vi "Main.vi"(11 "Module Admin":refnum<class "Delacor_lib_QMH_Cloneable Module Admin.lvclass">) -> ()   [LabVIEW 2020, in "TDS1002 Oscilloscope.lvlib"]
doc: "This template is based off of the Queued Message Handler design pattern and the Queued Message Handler project template that ships with LabVIEW.\n\nThe main difference is that the queue is private to this module and communication between modules is performed via Broadcast and Request events.\n\nRequest events are wrapped in public API methods and are handled in the Event Handling Loop (EHL) of this VI. Any module can register for Broadcast events sent by this module. The EHL generates messages based on user interface actions.\n\nThe Message Handling Loop (MHL) processes messages generated by the EHL, or by other messages. The messages are string values, so new messages can be added easily to the Message Cases case structure in the MHL. Each message cluster can also provide an optional value for Message Data, which is a variant that can be converted to whatever message-specific data is required.\n_____\nBased on DQMH Project Template 6.1.0.94.\n____\nPantherLAB Templates 1.0.0.1\nCopyright (c) 2022, PantherLAB\n____\nPantherLAB Templates 1.0.0.5\nCopyright (c) 2022, PantherLAB"
uses:
  TDS1002 Oscilloscope.lvlib
  <vilib>/Delacor/Delacor QMH/Libraries/Cloneable Module Admin_class/Delacor_lib_QMH_Cloneable Module Admin.lvclass
  C:/Program Files (x86)/National Instruments/LabVIEW 2020/vi.lib/Delacor/Delacor QMH/Libraries/Module Admin_class/Delacor_lib_QMH_Module Admin.lvclass
  Module Data--cluster.ctl
  <vilib>/Delacor/Delacor QMH/Libraries/Cloneable Module Admin_class/Delacor_lib_QMH_Cloneable Module Admin.lvclass/Delacor_lib_QMH_Cloneable Module Admin.ctl
  Helper Loop Status--enum.ctl
  <vilib>/Delacor/Delacor QMH/Libraries/Message Queue_class/Delacor_lib_QMH_Message Queue.lvclass/Delacor_lib_QMH_Message Queue.ctl
  Stop Argument--cluster.ctl
  <vilib>/Delacor/Delacor QMH/Libraries/Module Admin_class/Delacor_lib_QMH_Module Admin.lvclass/Delacor_lib_QMH_Module Admin.ctl
  Draw Panel into Subpanel Argument--cluster.ctl
  Remove Panel from Subpanel Argument--cluster.ctl
  Connect Argument--cluster.ctl
  Disconnect Argument--cluster.ctl
  Configure acquisition Argument--cluster.ctl
  Support/Channel configuration--cluster.ctl
  Configure trigger Argument--cluster.ctl
  Trigger config--cluster.ctl
  Send software trigger Argument--cluster.ctl
  Start continuous acquistion Argument--cluster.ctl
  Stop continuous acquisition Argument--cluster.ctl
  Get measurement Argument--cluster.ctl
  Get measurement (Reply Payload)--cluster.ctl
  Configure timebase Argument--cluster.ctl
  <vilib>/Utility/miscctls.llb/LVPointTypeDef.ctl
  Helper loop arguments--cluster.ctl
  <vilib>/Delacor/Delacor QMH/Libraries/Cloneable Module Admin_class/Delacor_lib_QMH_Get Module ID.vi
  <vilib>/Delacor/Delacor QMH/Libraries/Message Queue_class/Delacor_lib_QMH_Enqueue Message (Single).vi
  <vilib>/Delacor/Delacor QMH/Libraries/Module Admin_class/Delacor_lib_QMH_Get External Launch.vi
  <instrlib>/Tektronix TDS 200 1000 2000 Series/Public/Data/Read (Single Waveform).vi
  <instrlib>/Tektronix TDS 200 1000 2000 Series/Public/Configure/Configure Trigger (Edge).vi
  <vilib>/Utility/error.llb/Error Cluster From Error Code.vi
  <vilib>/ErrorRing/Error Ring.xnode
  <vilib>/Delacor/Delacor QMH/Libraries/Message Queue_class/Delacor_lib_QMH_Message Queue.lvclass
  Local Events/Local Events.lvlib
  <instrlib>/Tektronix TDS 200 1000 2000 Series/Tektronix TDS 200 1000 2000 Series.lvlib
panel:
  out "Waveform Data":waveform(dbl)(graph)
  out "error out":errorcluster
  out "Status":string
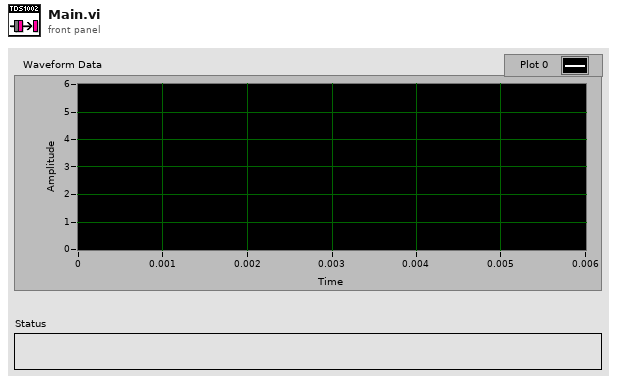
[diagram p1: front panel]
types:
  T1 = typedef "TDS1002 Oscilloscope.lvlib/Request Events--cluster.ctl" = cluster{"Stop Module":refnum<user-event>, "Show Panel":refnum<user-event>, "Hide Panel":refnum<user-event>, "Show Diagram":refnum<user-event>, "Get Module Execution Status":refnum<user-event>, "Draw Panel into Subpanel":refnum<user-event>, "Remove Panel from Subpanel":refnum<user-event>, "Connect":refnum<user-event>, "Disconnect":refnum<user-event>, "Configure acquisition":refnum<user-event>, "Configure trigger":refnum<user-event>, "Send software trigger":refnum<user-event>, "Start continuous acquistion":refnum<user-event>, "Stop continuous acquisition":refnum<user-event>, "Get measurement":refnum<user-event>, "Configure timebase":refnum<user-event>}
  T2 = typedef "TDS1002 Oscilloscope.lvlib/Local Events.lvlib/Local Events--cluster.ctl" = cluster{"Wake up Helper Loop":refnum<user-event>, "Put Helper Loop to Sleep":refnum<user-event>}
  T3 = typedef "TDS1002 Oscilloscope.lvlib/Module Data--cluster.ctl" = cluster{"Status":string, "SubPanel":refnum<vi>, "Panel Status":bool, "VISA resource":refnum<visa-resource-name>, "Acquisition type":enum16{"On demand", "Continous"}}
  T4 = typedef "TDS1002 Oscilloscope.lvlib/Helper Loop Status--enum.ctl" = enum16{"Awake", "Asleep"}
  T5 = enum32{"invalid lock state", "Not Locked", "Locked (No Password)", "Password-protected"}
  T6 = typedef "TDS1002 Oscilloscope.lvlib/Stop Argument--cluster.ctl" = cluster{"Module ID":i32, "Origin":string, "Exit via Stop Module Req?":bool, "Wait for Module to stop?":bool}
  T7 = typedef "TDS1002 Oscilloscope.lvlib/Draw Panel into Subpanel Argument--cluster.ctl" = cluster{"Module ID":i32, "Sub Panel":refnum<vi>}
  T8 = typedef "TDS1002 Oscilloscope.lvlib/Remove Panel from Subpanel Argument--cluster.ctl" = cluster{"Module ID":i32, "Boolean":bool}
  T9 = typedef "TDS1002 Oscilloscope.lvlib/Connect Argument--cluster.ctl" = cluster{"Module ID":i32, "VISA resource":refnum<visa-resource-name>}
  T10 = typedef "TDS1002 Oscilloscope.lvlib/Disconnect Argument--cluster.ctl" = cluster{"Module ID":i32, "Boolean":bool}
  T11 = typedef "TDS1002 Oscilloscope.lvlib/Configure acquisition Argument--cluster.ctl" = cluster{"Module ID":i32, "Acquisition type":enum16{"On demand", "Continous"}, "Config parameters":T12}
  T12 = typedef "TDS1002 Oscilloscope.lvlib/Channel configuration--cluster.ctl" = cluster{"Acquisition Type":i32, "Averaged Waveforms":i32, "Channel":i32, "Probe Attenuation":i32, "Timebase":dbl}
  T13 = typedef "TDS1002 Oscilloscope.lvlib/Configure trigger Argument--cluster.ctl" = cluster{"Module ID":i32, "Trigger config":T14}
  T14 = typedef "TDS1002 Oscilloscope.lvlib/Trigger config--cluster.ctl" = cluster{"Trigger Source":i32, "Trigger Mode":i32, "Trigger Slope":i32, "Trigger Coupling":i32, "Trigger Level":dbl}
  T15 = typedef "TDS1002 Oscilloscope.lvlib/Send software trigger Argument--cluster.ctl" = cluster{"Module ID":i32, "Boolean":bool}
  T16 = typedef "TDS1002 Oscilloscope.lvlib/Start continuous acquistion Argument--cluster.ctl" = cluster{"Module ID":i32, "Timeout":i32}
  T17 = typedef "TDS1002 Oscilloscope.lvlib/Stop continuous acquisition Argument--cluster.ctl" = cluster{"Module ID":i32, "Boolean":bool}
  T18 = typedef "TDS1002 Oscilloscope.lvlib/Get measurement Argument--cluster.ctl" = cluster{"Module ID":i32, "Channel":i32, "Measurement Type":i32, "Wait Notifier":refnum<notifier>, "wait for reply":bool}
  T19 = typedef "TDS1002 Oscilloscope.lvlib/Configure timebase Argument--cluster.ctl" = cluster{"Module ID":i32, "Timebase":dbl}
  T20 = typedef "LVPointTypeDef.ctl" = cluster{"Horizontal":i16, "Vertical":i16}
  T21 = enum32{"Invalid", "Standard", "Closed", "Hidden", "Minimized", "Maximized"}
  T22 = cluster{"Baud Rate":u32, "Parity":u16, "Stop Bits":u16, "Flow Control":u16}
  T23 = typedef "TDS1002 Oscilloscope.lvlib/Helper loop arguments--cluster.ctl" = cluster{"Helper Loop Timeout":i32, "VISA resource name":refnum<visa-resource-name>}
  T24 = typedef "TDS1002 Oscilloscope.lvlib/Get measurement (Reply Payload)--cluster.ctl" = cluster{"Value":dbl, "error":errorcluster}
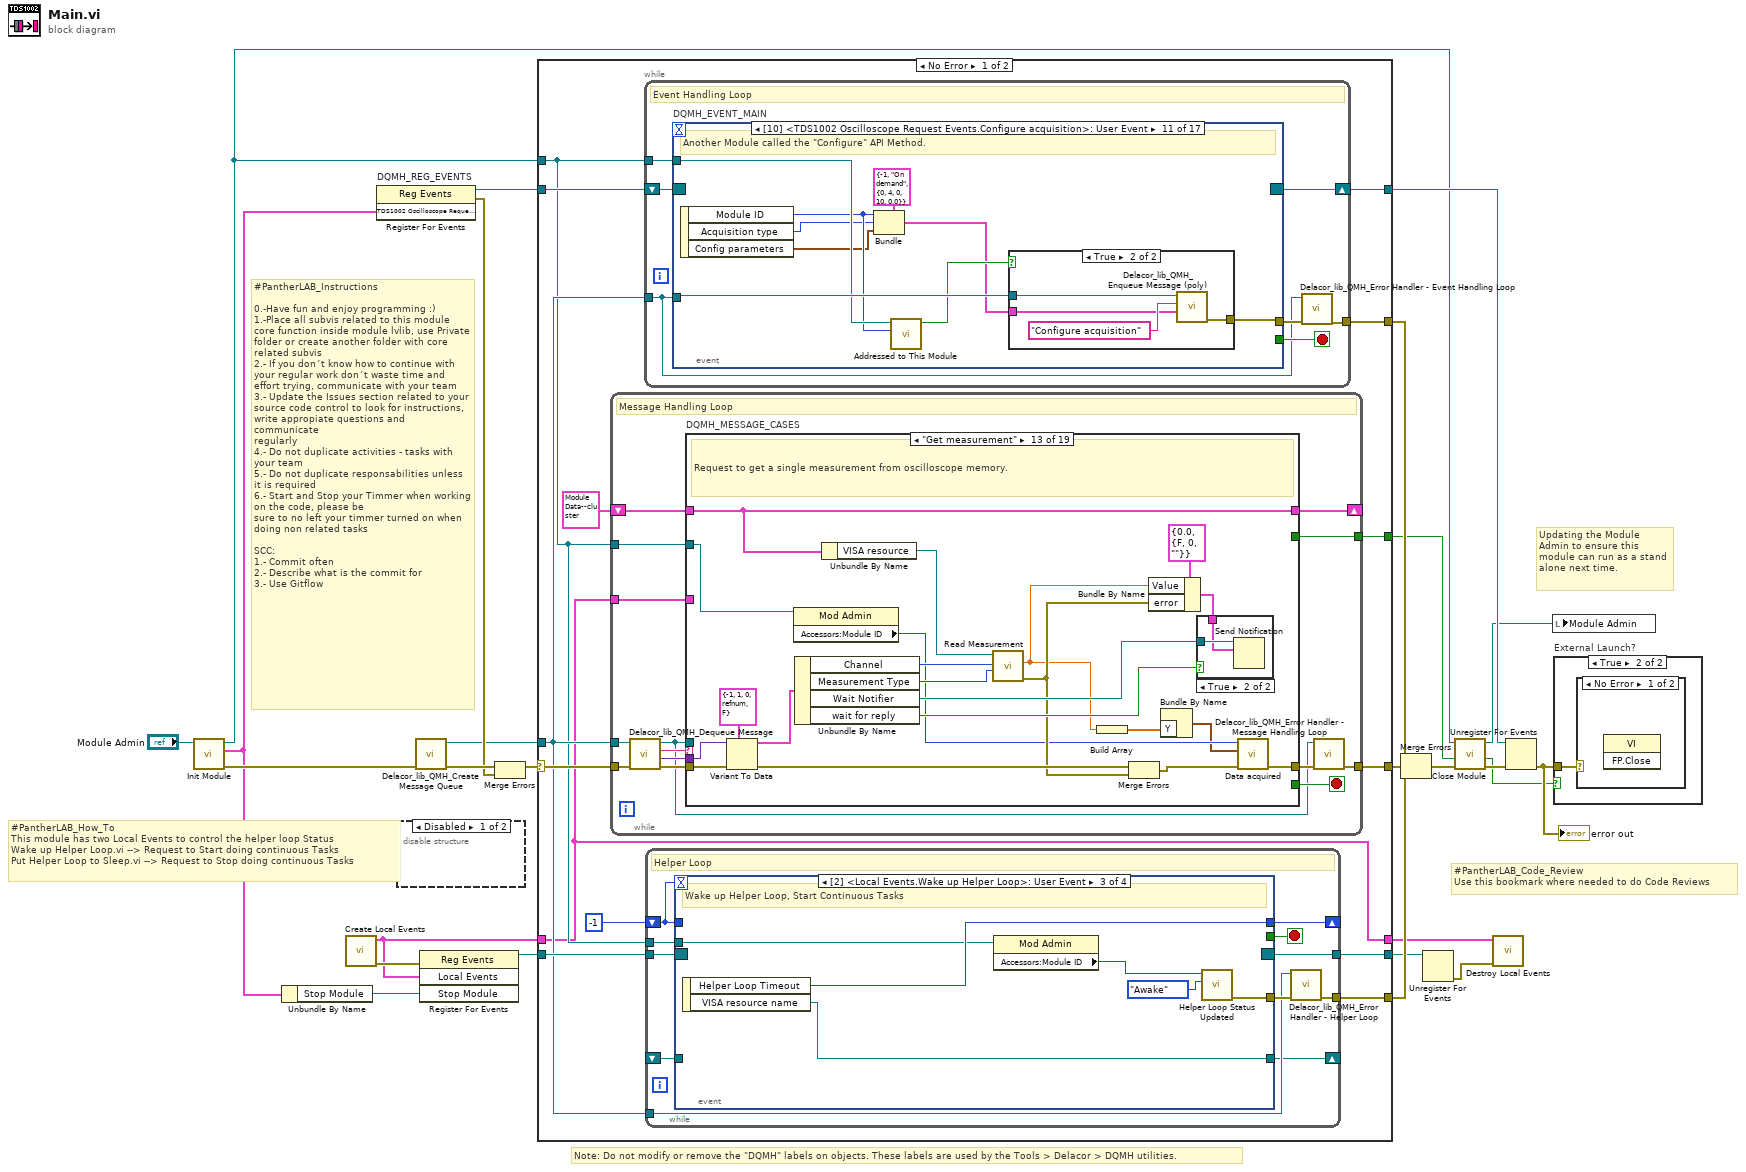
[diagram p0: block diagram]
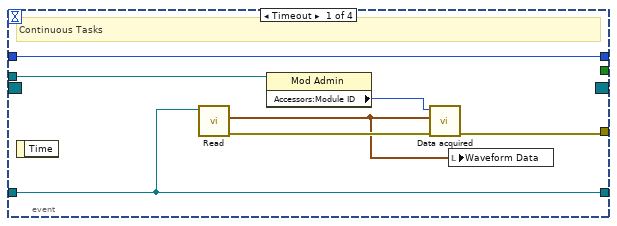
[diagram p3: hidden frame]
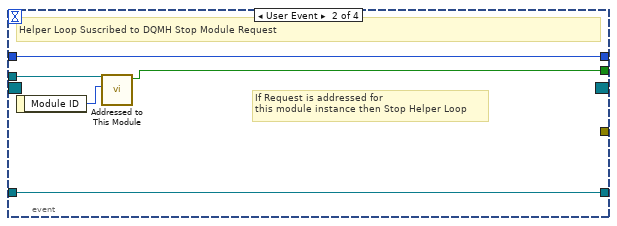
[diagram p4: hidden frame]
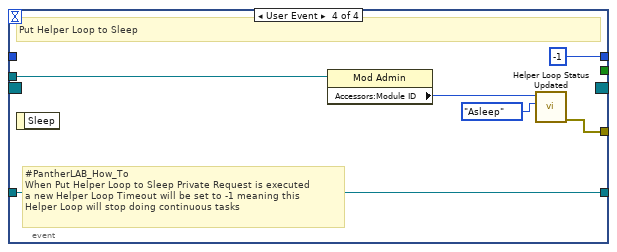
[diagram p5: hidden frame]
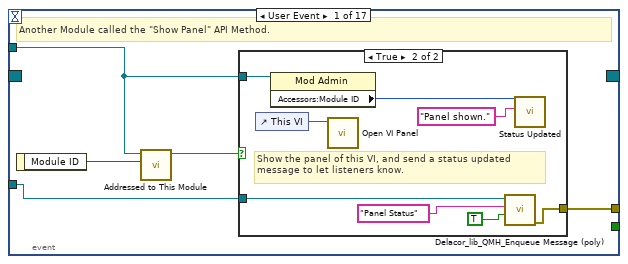
[diagram p6: hidden frame]
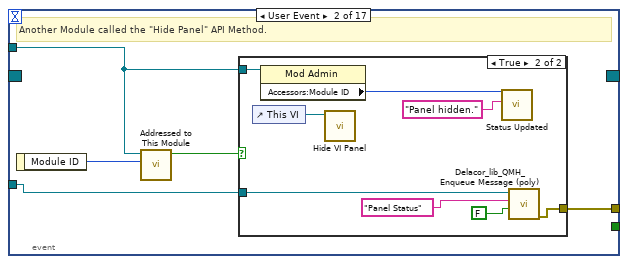
[diagram p8: hidden frame]
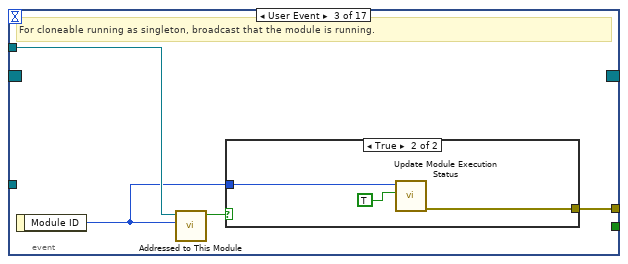
[diagram p10: hidden frame]
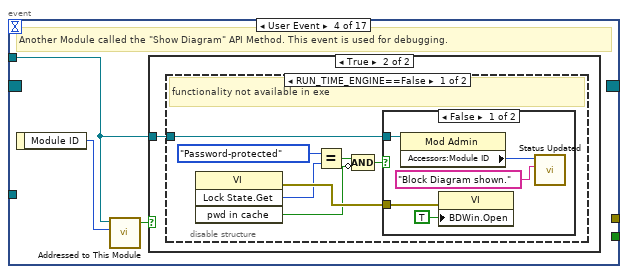
[diagram p12: hidden frame]
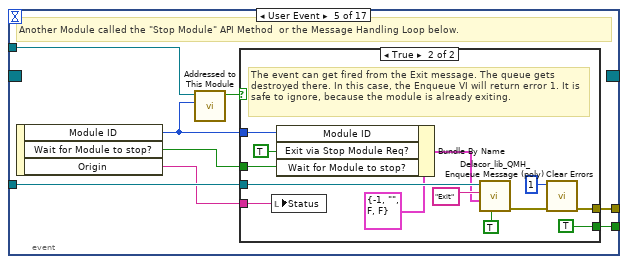
[diagram p16: hidden frame]
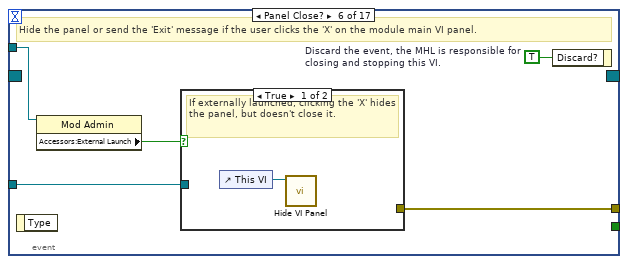
[diagram p18: hidden frame]
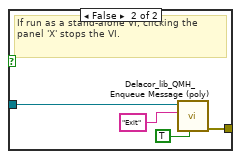
[diagram p19: hidden frame]
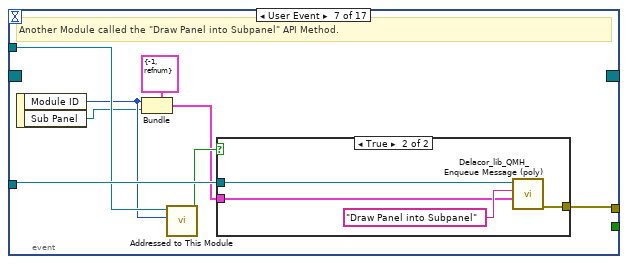
[diagram p20: hidden frame]
diagram:
  # "#PantherLAB_How_To\nThis module has two Local Events to control the helper loop Status\nWake up Helper Loop.vi --> Request to Start doing continuous Tasks\nPut Helper Loop to Sleep.vi --> Request to Stop doing continuous Tasks"
  # "#PantherLAB_Code_Review\nUse this bookmark where needed to do Code Reviews"
  # "#PantherLAB_Instructions\n\n0.-Have fun and enjoy programming :)\n1.-Place all subvis related to this module core function inside module lvlib, use Private folder or create another folder with core related subvis \n2.- If you don´t know how to continue with your regular work don´t waste time and effort trying, communicate with your team\n3.- Update the Issues section related to your source code control to look for instructions, write appropiate questions and communicate\nregularly\n4.- Do not duplicate activities - tasks with your team\n5.- Do not duplicate responsabilities unless it is required\n6.- Start and Stop your Timmer when working on the code, please be\nsure to no left your timmer turned on when doing non related tasks\n\nSCC:\n1.- Commit often\n2.- Describe what is the commit for\n3.- Use Gitflow"
  # "Note: Do not modify or remove the \"DQMH\" labels on objects. These labels are used by the Tools > Delacor > DQMH utilities."
  # "Updating the Module Admin to ensure this module can run as a stand alone next time."
  n1 = call "Init Module.vi"("Cloneable Module Admin in"="Module Admin") -> ("error out"=w23:errorcluster, "TDS1002 Oscilloscope Request Events"=w4:T1, "Cloneable Module Admin out"=w10:refnum<class "Delacor_lib_QMH_Cloneable Module Admin.lvclass">)  [unwired: 8 in]
  n2 = Unbundle By Name(w4) -> ("Stop Module"=w3:refnum<user-event>)
  n3 = call "Create Local Events.vi"() -> ("error out"=w16:errorcluster, "Local Events"=w2:T2)  [unwired: 10 in]
  n4 = register-events "DQMH_REG_EVENTS"(w4) -> (reference out=w13:refnum<event-registration>, error out=w18:errorcluster)  [unwired: 2 in]
  n5 = disable-structure shown="Disabled" {
    frame Disabled {
    }
    frame Enabled {
    }
  }
  n6 = call <vilib>:"Delacor_lib_QMH_Create Message Queue.vi"("error in"=w23) -> ("error out"=w20:errorcluster, "Message Queue"=w12:refnum<class "Delacor_lib_QMH_Message Queue.lvclass">)  [unwired: 9 in]
  n7 = register-events(error in=w16, w2, w3) -> (reference out=w5:refnum<event-registration>)  [unwired: 1 in, 1 out]
  n8 = Merge Errors(w20, w18) -> (w19:errorcluster)
  n9 = case shown="No Error" w19 {
    selector: w19 -> [w38 w577]
    tunnel: [w40 w576] -> w24
    tunnel: [w36 w575] -> w14
    tunnel: w13 -> [w34 w575]
    tunnel: w12 -> [w29 w568]
    tunnel: [w39 _] -> w25
    tunnel: w10 -> [w28 w571]
    tunnel: [w33 _] -> w8
    tunnel: [w32 w567] -> w6
    tunnel: w5 -> [w31 w567]
    tunnel: [w37 _] -> w17
    tunnel: w2 -> [w27 w566]
    tunnel: [w27 w566] -> w1
    frame No Error {
      n10 = while {
        tunnel: w29 -> [w303]
        shift-right: [w307] -> _
        shift-left: T3 {"Status"="", "SubPanel"=refnum, "Panel Status"=FALSE, "VISA resource"="", "Acquisition type"=enum."On demand"} ("Data Cluster") -> [w308]
        tunnel: w38 -> [w311]
        tunnel: [w309] -> w40
        tunnel: w28 -> [w301]
        tunnel: [w300] -> w33
        tunnel: w27 -> [w299]
        stop <- w306 stop-if-true
        # "Message Handling Loop"
        n11 = call-dynamic "Delacor_lib_QMH_Dequeue Message.vi"("error in"=w311, "Message Queue in"=w303) -> ("error out"=w310:errorcluster, "Message Data"=w304:variant, "Message"=w305:string, "Message Queue out"=w302:refnum<class "Delacor_lib_QMH_Message Queue.lvclass">)  [unwired: 6 in]
        n12 = case "DQMH_MESSAGE_CASES" shown="\"Get measurement\"" w305 {
          selector: w305 -> [_ _ _ _ _ _ _ _ _ _ _ _ _ _ _ _ _ _ w553]
          tunnel: w302 -> [_ _ _ _ _ _ _ _ _ _ _ _ _ _ _ _ w517 w543 _]
          tunnel: w310 -> [w331 w335 w342 w354 w373 w398 w409 w424 w440 w458 w470 w478 w499 w510 w513 w515 w526 w549 w555]
          tunnel: [w329 w335 w341 w352 w372 w385 w401 w411 w426 w445 w465 w472 w484 w505 w512 w515 w522 w546 w556] -> w312
          tunnel: w308 -> [w322 w334 w340 w345 w367 w391 w404 w418 w435 w453 w462 w477 w490 w503 w511 w514 w521 w534 w554]
          tunnel: [w321 w334 w337 w344 w367 w389 w404 w416 w435 w453 w462 w477 w490 w503 w511 w514 w521 w534 w554] -> w307
          tunnel: [_ _ _ _ _ _ _ _ _ _ _ _ _ _ _ _ _ w542 _] -> w306
          tunnel: w304 -> [_ _ w339 w350 w371 w397 w408 w423 w439 w457 w469 w476 w497 w509 _ _ w520 w540 _]
          tunnel: w301 -> [w316 _ _ w343 w366 w388 w400 w413 _ w447 _ _ w483 _ _ _ w519 w536 w551]
          tunnel: [_ _ _ _ _ _ _ _ _ _ _ _ _ _ _ _ _ w538 _] -> w300
          tunnel: w299 -> [_ _ _ _ _ _ _ _ _ _ w464 w471 _ _ _ _ _ _ _]
          frame "Initialize" {
            w313 = "Initial Message" ("Initial Message")
            # "#CodeNeeded - Initialize the appearance of the front panel."
            # "#CodeNeeded - Initialize your state data here."
            # "Initialize - Any operation that needs to be done before the module can receive messages. Synchronize Caller Events.vi will inform Start Module.vi that the module has launched and is ready to receive messages. Module Did Init.vi will broadcast that the module initialized."
            n13 = call "Synchronize Caller Events.vi"("error in (no error)"=w331, "Module Admin"=w316) -> ("error out"=w330:errorcluster, "Module Admin out"=w315:refnum<class "Delacor_lib_QMH_Cloneable Module Admin.lvclass">)  [unwired: 8 in]
            n14 = property class="Mod Admin"(reference=w315) -> ("Accessors:Module ID"=w318:i32, "Accessors:External Launch"=w317:bool)  [unwired: 1 in, 2 out]
            n15 = call "Module Name--constant.vi"("Module ID"=w318) -> ("Module Name"=w326:string)  [unwired: 10 in]
            n16 = property class="VI"("Front Panel.Title"=w326) -> (reference out=w328:refnum<vi>, error out=w333:errorcluster)  [unwired: 2 in]
            n17 = Select(t=T21."Hidden" ("State"), s=w317, f=T21."Standard" ("State")) -> (s? t:f=w323:T21)
            n18 = invoke class="VI" method="FP.Open"(reference=w328, error in=w333, "State"=w323) -> (reference out=w327:refnum<vi>, error out=w332:errorcluster)  [unwired: 2 in, 3 out]
            n19 = call "Module Name--constant.vi"("Module ID"=w318) -> ("Module Name"=w319:string)  [unwired: 10 in]
            n20 = Bundle By Name(cluster=w322, "Status"=w313) -> (w321:T3)
            n21 = invoke class="VI" method="FP.Center"(reference=w327, error in=w332) -> ()  [unwired: 1 in, 3 out]
            n22 = property on="Pane" class="Pane"("Origin"=T20 {"Horizontal"=0, "Vertical"=0}) -> ()  [unwired: 2 in, 2 out]
            n23 = call "Module Did Init.vi"("error in (no error)"=w330, "Initialized?"=TRUE, "Origin"=w319, "Module ID"=w318) -> ("error out"=w329:errorcluster)  [unwired: 7 in]
            "Status" <- w313
          }
          frame "---Module Specific---" {
            # "Separator -- The following cases handle messages specific to this Module."
          }
          frame "Panel Status" {
            n24 = Variant To Data(error in=w342, type=TRUE, Variant=w339) -> (data=w336:bool, error out=w341:errorcluster)
            n25 = Bundle By Name(cluster=w340, "Panel Status"=w336) -> (w337:T3)
          }
          frame "Draw Panel into Subpanel" {
            # "Draw instance panel into panel provided"
            n26 = Variant To Data(error in=w354, type=T7 {"Module ID"=-1, "Sub Panel"=refnum} ("Draw Panel into Subpanel Argument"), Variant=w350) -> (data=w348:T7, error out=w353:errorcluster)
            n27 = Unbundle By Name(w348) -> ("Module ID"=w346:i32, "Sub Panel"=w347:refnum<vi>)
            n28 = case shown="Default" w346 {
              tunnel: w347 -> [_ w364]
              tunnel: [w359 w365] -> w351
              tunnel: w345 -> [w357 w362]
              tunnel: [w357 w361] -> w344
              tunnel: w343 -> [w356 _]
              frame Default {
                n29 = property class="Mod Admin"(reference=w356) -> ("Accessors:Module ID"=w355:i32)  [unwired: 1 in, 2 out]
                n30 = call "Status Updated.vi"("Status"="Please send \"Draw Panel into Subpanel\" Request to this Module ID Instance", "Module ID"=w355) -> ("error out"=w359:errorcluster)  [unwired: 9 in]
              }
              frame 0.. {
                n31 = control-ref of="This VI"() -> (w363:refnum<vi>)
                n32 = call "Draw Panel into Subpanel Procedure.vi"("SubPanel in"=w364, "This VI"=w363) -> ("error out"=w365:errorcluster, "SubPanel out"=w360:refnum<vi>)  [unwired: 8 in]
                n33 = Bundle By Name(cluster=w362, "SubPanel"=w360) -> (w361:T3)
              }
            }
            n34 = Merge Errors(w353, w351) -> (w352:errorcluster)
          }
          frame "Remove Panel from Subpanel" {
            # "Remove panel from subpanel"
            n35 = Variant To Data(error in=w373, type=T8 {"Module ID"=-1, "Boolean"=FALSE} ("Remove Panel from Subpanel Argument"), Variant=w371) -> (data=w369:T8, error out=w372:errorcluster)
            n36 = Unbundle By Name(w369) -> ("Module ID"=w368:i32)
            n37 = case shown="-1" w368 {
              tunnel: w367 -> [w377 _]
              tunnel: w366 -> [_ w381]
              frame Default {
                n38 = Unbundle By Name(w377) -> ("Panel Status"=w375:bool, "SubPanel"=w376:refnum<vi>)
                n39 = control-ref of="This VI"() -> (w374:refnum<vi>)
                n40 = case shown="True" w375 {
                  tunnel: w374 -> [w378 w379]
                  frame False {
                    n41 = call "Hide VI Panel.vi"("VI"=w378) -> ()  [unwired: 10 in, 1 out]
                  }
                  frame True {
                    n42 = call "Open VI Panel.vi"("VI"=w379) -> ()  [unwired: 10 in, 1 out]
                  }
                }
                n43 = invoke class="SubPnl" method="Remove VI"(reference=w376) -> ()  [unwired: 2 in, 3 out]
              }
              frame -1 {
                n44 = property class="Mod Admin"(reference=w381) -> ("Accessors:Module ID"=w380:i32)  [unwired: 1 in, 2 out]
                n45 = call "Status Updated.vi"("Status"="Please send \"Remove panel from subpanel\" Request to this Module ID Instance", "Module ID"=w380) -> ()  [unwired: 9 in, 1 out]
              }
            }
          }
          frame "Connect" {
            w383 = FALSE  # ID Query?
            w384 = FALSE  # Reset?
            # "Request to connect to a given TDS1000 series oscilloscope."
            n46 = Variant To Data(error in=w398, type=T9 {"Module ID"=-1, "VISA resource"=""} ("Connect Argument"), Variant=w397) -> (data=w395:T9, error out=w394:errorcluster)
            n47 = Unbundle By Name(w395) -> ("VISA resource"=w393:refnum<visa-resource-name>)  [unwired: 1 out]
            n48 = property class="Mod Admin"(reference=w388) -> ("Accessors:Module ID"=w387:i32)  [unwired: 1 in, 2 out]
            n49 = call <instrlib>:"Initialize.vi"("Serial Configuration"=T22 {"Baud Rate"=9600, "Parity"=0, "Stop Bits"=10, "Flow Control"=2}, "error in (no error)"=w394, "Reset? (T: Yes)"=w384, "ID Query? (T: Yes)"=w383, "VISA resource name"=w393) -> ("error out"=w386:errorcluster, "VISA resource name out"=w390:refnum<visa-resource-name>)  [unwired: 5 out]
            n50 = Bundle By Name(cluster=w391, "VISA resource"=w390) -> (w389:T3)
            n51 = call "Device connected.vi"("error in"=w386, "Module ID"=w387) -> ("error out"=w385:errorcluster)  [unwired: 9 in]
          }
          frame "Disconnect" {
            # "Request to disconnect from the device."
            n52 = Variant To Data(error in=w409, type=T10 {"Module ID"=-1, "Boolean"=FALSE} ("Disconnect Argument"), Variant=w408) -> (data=w406:T10, error out=w405:errorcluster)
            n53 = Unbundle By Name(w406) -> ()  [unwired: 2 out]
            n54 = Unbundle By Name(w404) -> ("VISA resource"=w403:refnum<visa-resource-name>)
            n55 = call <instrlib>:"Close.vi"("error in (no error)"=w405, "VISA resource name"=w403) -> ("error out"=w402:errorcluster)  [unwired: 9 out]
            n56 = property class="Mod Admin"(reference=w400) -> ("Accessors:Module ID"=w399:i32)  [unwired: 1 in, 2 out]
            n57 = call "Device disconnected.vi"("error in"=w402, "Module ID"=w399) -> ("error out"=w401:errorcluster)  [unwired: 9 in]
          }
          frame "Configure acquisition" {
            # "Request to configure the acquisition parameters."
            n58 = Variant To Data(error in=w424, type=T11 {"Module ID"=-1, "Acquisition type"=enum."On demand", "Config parameters"={"Acquisition Type"=0, "Averaged Waveforms"=4, "Channel"=0, "Probe Attenuation"=10, "Timebase"=0.0}} ("Configure Argument"), Variant=w423) -> (data=w421:T11, error out=w420:errorcluster)
            n59 = Unbundle By Name(w421) -> ("Config parameters"=w415:T12, "Acquisition type"=w414:enum16{"On demand", "Continous"})
            n60 = Unbundle By Name(w418) -> ("VISA resource"=w419:refnum<visa-resource-name>)
            n61 = property class="Mod Admin"(reference=w413) -> ("Accessors:Module ID"=w410:i32)  [unwired: 1 in, 2 out]
            n62 = call "Configure acquisition--VISA.vi"("error in (no error)"=w420, "Type"=w414, "Config parameters"=w415, "VISA Refnum in"=w419) -> ("error out"=w412:errorcluster, "VISA resource name out"=w417:refnum<visa-resource-name>)  [unwired: 6 in]
            n63 = Bundle By Name(cluster=w418, "VISA resource"=w417, "Acquisition type"=w414) -> (w416:T3)
            n64 = call "Configuration applied.vi"("error in"=w412, "Module ID"=w410) -> ("error out"=w411:errorcluster)  [unwired: 9 in]
          }
          frame "Configure trigger" {
            # "Request to configure the trigger of a pre-configured channel."
            n65 = Unbundle By Name(w435) -> ("Acquisition type"=w427:enum16{"On demand", "Continous"}, "VISA resource"=w434:refnum<visa-resource-name>)
            n66 = Variant To Data(error in=w440, type=T13 {"Module ID"=-1, "Trigger config"={"Trigger Source"=0, "Trigger Mode"=0, "Trigger Slope"=0, "Trigger Coupling"=0, "Trigger Level"=0.0}} ("Configure trigger Argument"), Variant=w439) -> (data=w437:T13, error out=w436:errorcluster)
            n67 = Unbundle By Name(w437) -> ("Trigger config.Trigger Source"=w433:i32, "Trigger config.Trigger Level"=w432:dbl, "Trigger config.Trigger Mode"=w431:i32, "Trigger config.Trigger Slope"=w430:i32, "Trigger config.Trigger Coupling"=w429:i32)
            n68 = call-poly <instrlib>:"Configure Trigger.vi"("VISA resource name"=w434, "Trigger Source (0: Channel 1)"=w433, "Trigger Level (0.0 V)"=w432, "Trigger Mode (0: Auto)"=w431, "error in (no error)"=w436, "Trigger Slope (0: Rising)"=w430, "Trigger Coupling (0: AC)"=w429) -> ("VISA resource name out"=w425:refnum<visa-resource-name>, "error out"=w428:errorcluster)  [unwired: 7 in]
            n69 = case shown="\"On demand\", Default" w427 {
              tunnel: w428 -> [w443 w444]
              tunnel: [w442 w444] -> w426
              tunnel: w425 -> [w441 _]
              frame "On demand", Default {
                n70 = call <instrlib>:"Wait for Trigger.vi"("error in (no error)"=w443, "VISA resource name"=w441) -> ("error out"=w442:errorcluster)  [unwired: 8 in, 1 out]
              }
              frame "Continous" {
              }
            }
          }
          frame "Send software trigger" {
            # "Request to send a software trigger."
            n71 = Unbundle By Name(w453) -> ("VISA resource"=w452:refnum<visa-resource-name>)
            n72 = Variant To Data(error in=w458, type=T15 {"Module ID"=-1, "Boolean"=FALSE} ("Send software trigger Argument"), Variant=w457) -> (data=w455:T15, error out=w454:errorcluster)
            n73 = Unbundle By Name(w455) -> ()  [unwired: 1 out]
            n74 = call <instrlib>:"Send Software Trigger.vi"("error in (no error)"=w454, "VISA resource name"=w452) -> ("error out"=w451:errorcluster, "VISA resource name out"=w450:refnum<visa-resource-name>)  [unwired: 8 in]
            n75 = call-poly <instrlib>:"Read.vi"("error in (no error)"=w451, "VISA resource name"=w450) -> ("error out"=w449:errorcluster, "Waveform Data"=w448:waveform(dbl))  [unwired: 7 in, 1 out]
            "Waveform Data" <- w448
            n76 = property class="Mod Admin"(reference=w447) -> ("Accessors:Module ID"=w446:i32)  [unwired: 1 in, 2 out]
            n77 = call "Data acquired.vi"("error in"=w449, "Waveform"=w448, "Module ID"=w446) -> ("error out"=w445:errorcluster)  [unwired: 8 in]
          }
          frame "Start continuous acquistion" {
            # "Request to start continuous acquisition."
            n78 = Variant To Data(error in=w470, type=T16 {"Module ID"=-1, "Timeout"=0} ("Start continuous acquistion Argument"), Variant=w469) -> (data=w467:T16, error out=w466:errorcluster)
            n79 = Unbundle By Name(w462) -> ("VISA resource"=w461:refnum<visa-resource-name>)
            n80 = Unbundle By Name(w467) -> ("Timeout"=w460:i32)
            n81 = Bundle By Name(cluster=T23 {"Helper Loop Timeout"=0, "VISA resource name"=""}, "VISA resource name"=w461, "Helper Loop Timeout"=w460) -> (w459:T23)
            n82 = call "Wake up Helper Loop.vi"("error in"=w466, "HL Arguments"=w459, "Local Events"=w464) -> ("error out"=w465:errorcluster)  [unwired: 8 in]
          }
          frame "Stop continuous acquisition" {
            # "Request to stop continuous aquisition."
            n83 = Variant To Data(error in=w478, type=T17 {"Module ID"=-1, "Boolean"=FALSE} ("Stop continuous acquisition Argument"), Variant=w476) -> (data=w474:T17, error out=w473:errorcluster)
            n84 = Unbundle By Name(w474) -> ()  [unwired: 1 out]
            n85 = call "Put Helper Loop to Sleep.vi"("error in"=w473, "Local Events"=w471) -> ("error out"=w472:errorcluster)  [unwired: 9 in]
          }
          frame "Get measurement" {
            # "Request to get a single measurement from oscilloscope memory."
            n86 = Variant To Data(error in=w499, type=T18 {"Module ID"=-1, "Channel"=1, "Measurement Type"=0, "Wait Notifier"=refnum, "wait for reply"=FALSE} ("Get measurement Argument"), Variant=w497) -> (data=w495:T18, error out=w498:errorcluster)
            n87 = property class="Mod Admin"(reference=w483) -> ("Accessors:Module ID"=w482:i32)  [unwired: 1 in, 2 out]
            n88 = Unbundle By Name(w495) -> ("Channel"=w488:i32, "Measurement Type"=w487:i32, "Wait Notifier"=w494:refnum<notifier>, "wait for reply"=w493:bool)
            n89 = Unbundle By Name(w490) -> ("VISA resource"=w489:refnum<visa-resource-name>)
            n90 = call <instrlib>:"Read Measurement.vi"("Measurement Type (0: Frequency)"=w487, "Channel (1: Channel 1)"=w488, "VISA resource name"=w489) -> ("error out"=w486:errorcluster, "Measurement"=w481:dbl)  [unwired: 5 in, 2 out]
            n91 = Build Array(w481) -> (w480:dbl[])
            n92 = Merge Errors(w498, w486) -> (w485:errorcluster)
            n93 = Bundle By Name(cluster=T24 {"Value"=0.0, "error"={"status"=FALSE, "code"=0, "source"=""}} ("Get measurement (Reply Payload)"), "Value"=w481, "error"=w486) -> (w492:T24)
            n94 = Bundle By Name("Y"=w480) -> (w479:waveform(dbl))  [unwired: 1 in]
            n95 = case shown="True" w493 {
              tunnel: w494 -> [_ w501]
              tunnel: w492 -> [_ w500]
              frame False {
              }
              frame True {
                n96 = Send Notification(notification=w500, notifier=w501) -> ()  [unwired: 1 in, 2 out]
              }
            }
            n97 = call "Data acquired.vi"("error in"=w485, "Waveform"=w479, "Module ID"=w482) -> ("error out"=w484:errorcluster)  [unwired: 8 in]
          }
          frame "Configure timebase" {
            # "Request to configure the timebase of the oscilloscope."
            n98 = Variant To Data(error in=w510, type=T19 {"Module ID"=-1, "Timebase"=0.0005} ("Configure timebase Argument"), Variant=w509) -> (data=w507:T19, error out=w506:errorcluster)
            n99 = Unbundle By Name(w503) -> ("VISA resource"=w502:refnum<visa-resource-name>)
            n100 = Unbundle By Name(w507) -> ("Timebase"=w504:dbl)
            n101 = call <instrlib>:"Configure Timebase.vi"("error in (no error)"=w506, "Timebase (0.0005 s)"=w504, "VISA resource name"=w502) -> ("error out"=w505:errorcluster)  [unwired: 7 in, 1 out]
          }
          frame "---Copy This Frame---" {
            # "Duplicate this frame when creating new messages.  Change this comment in the duplicated frame to describe this message."
            n102 = Merge Errors(w513) -> (w512:errorcluster)
          }
          frame "---Exit and Error Handling---" {
            # "Separator - the following cases handle errors and exit messages."
          }
          frame "Error" {
            # "#CodeRecommended - If you ever change the name of this \"Error\" message, you'll need to update the name in the Check Loop Error.vi as well."
            # "#CodeRecommended - If the module is running in standalone mode (External Launch = FALSE), this code will pop up an error dialog and call the 'Exit' message if an error occurs. Add more fine-grained error handling here."
            # "Error - Check the error message data and respond accordingly. This message is sent by the \"Error Handler\" VIs at the end of each loop in this application."
            n103 = Variant To Data(error in=w526, type=errorcluster {"status"=FALSE, "code"=0, "source"=""} ("error constant"), Variant=w520) -> (data=w527:errorcluster, error out=w524:errorcluster)
            n104 = property class="Mod Admin"(reference=w519) -> ("Accessors:External Launch"=w518:bool, "Accessors:Module ID"=w516:i32)  [unwired: 1 in, 2 out]
            n105 = call "Error Reported.vi"("Error"=w527, "Module ID"=w516) -> ()  [unwired: 9 in, 1 out]
            n106 = case shown="False" w518 {
              tunnel: [w532 _] -> w523
              tunnel: w517 -> [w530 _]
              tunnel: w527 -> [w531 _]
              frame False {
                # "If the module is running standalone, then pop up an error dialog and call the \"Exit\" message."
                n107 = call <vilib>:"Simple Error Handler.vi"("error in (no error)"=w531) -> ()  [unwired: 4 in, 5 out]
                n108 = call-poly <vilib>:"Delacor_lib_QMH_Enqueue Message (poly).vi"("Priority Message? (F)"=TRUE, "Message"="Exit", "Message Queue in"=w530) -> ("error out"=w532:errorcluster)  [unwired: 7 in, 1 out]
              }
              frame True {
                # "If the module was launched externally, calling the Error Reported broadcast VI is the only action performed by the \"Error\" message. The module's caller can then process the error appropriately."
              }
            }
            n109 = Merge Errors(w524, w523) -> (w522:errorcluster)
            n110 = local write "error out"(w522) -> ()
          }
          frame "Exit" {
            w541 = 91  # 91: not all Exit messages will have an argument
            w542 = TRUE  # Stop the VI
            # "Release the message queue reference"
            # "Exit - Exit the application."
            n111 = Variant To Data(error in=w549, type=T6 {"Module ID"=-1, "Origin"="", "Exit via Stop Module Req?"=FALSE, "Wait for Module to stop?"=FALSE} ("Stop Argument"), Variant=w540) -> (data=w537:T6, error out=w544:errorcluster)
            n112 = call <vilib>:"Clear Errors.vi"("error in (no error)"=w544, "specific error code to clear (0: all)"=w541) -> ("error out"=w548:errorcluster)  [unwired: 4 in, 1 out]
            n113 = Unbundle By Name(w534) -> ("SubPanel"=w533:refnum<vi>)
            n114 = invoke class="SubPnl" method="Remove VI"(reference=w533) -> ()  [unwired: 2 in, 3 out]
            n115 = control-ref of="This VI"() -> (w535:refnum<vi>)
            n116 = call-dynamic "Delacor_lib_QMH_Release Message Queue.vi"("error in"=w548, "Message Queue"=w543) -> ("error out"=w547:errorcluster)  [unwired: 9 in]
            n117 = call "Handle Exit.vi"("Stop Argument"=w537, "Module Admin in"=w536, "VI reference"=w535) -> ("error out"=w545:errorcluster, "Wait for Stop?"=w538:bool)  [unwired: 7 in]
            n118 = Merge Errors(w547, w545) -> (w546:errorcluster)
          }
          frame Default {
            # "'Default' case only runs if there is a message that isn't defined in any of the other cases.  Output a programming error."
            n119 = property class="Mod Admin"(reference=w551) -> ("Accessors:Module ID"=w550:i32)  [unwired: 1 in, 2 out]
            n120 = call "Module Name--constant.vi"("Module ID"=w550) -> ("Module Name"=w552:string)  [unwired: 10 in]
            n121 = xnode "Error Ring"("parameter 0"=w553, "parameter 1"=w552) -> ("error out"=w557:errorcluster)
            n122 = Merge Errors(w555, w557) -> (w556:errorcluster)
          }
        }
        n123 = call-dynamic "Delacor_lib_QMH_Error Handler - Message Handling Loop.vi"("error in"=w312, "Message Queue in"=w302) -> ("dup error in"=w309:errorcluster)  [unwired: 8 in, 1 out]
      }
      n124 = while {
        tunnel: w29 -> [w76]
        shift-right: [w79] -> w36
        shift-left: w34 -> [w80]
        tunnel: [w81] -> w39
        tunnel: w28 -> [w77]
        stop <- w78 stop-if-true
        # "Event Handling Loop"
        n125 = event "DQMH_EVENT_MAIN" shown="[10] <TDS1002 Oscilloscope Request Events.Configure acquisition>: User Event" {
          selector: w80 -> [_ _ _ _ _ _ _ _ _ _ _ _ _ _ _ _ _]
          dyn-events: [_ _ _ _ _ _ _ _ _ _ _ _ _ _ _ _ _] -> w79
          timeout: _ -> [_ _ _ _ _ _ _ _ _ _ _ _ _ _ _ _ _]
          tunnel: [_ _ _ _ w135 _ _ _ _ _ _ _ _ _ _ _ _] -> w78
          tunnel: w76 -> [w83 w96 _ _ w138 w154 w169 w181 w194 w206 w219 w231 w243 w255 w267 w282 w294]
          tunnel: [w87 w100 w112 _ w139 w157 w170 w182 w187 w199 w213 w225 w236 w248 w260 w272 w287] -> w82
          tunnel: w77 -> [w84 w97 w110 w116 w137 w155 w167 w179 w192 w204 w217 w229 w241 w253 w265 w280 w292]
          event User Event {
            # "Another Module called the \"Show Panel\" API Method."
            n126 = event-data() -> ("Module ID"=w85:i32)  [unwired: 1 in]
            n127 = call "Addressed to This Module.vi"("Module ID from Argument"=w85, "Module Admin"=w84) -> ("Addressed to this instance?"=w86:bool)  [unwired: 8 in, 1 out]
            n128 = case shown="True" w86 {
              tunnel: w84 -> [_ w92]
              tunnel: w83 -> [_ w90]
              tunnel: [_ w95] -> w87
              frame False {
              }
              frame True {
                # "Show the panel of this VI, and send a status updated message to let listeners know."
                n129 = control-ref of="This VI"() -> (w94:refnum<vi>)
                n130 = property class="Mod Admin"(reference=w92) -> ("Accessors:Module ID"=w91:i32)  [unwired: 1 in, 2 out]
                n131 = call "Open VI Panel.vi"("VI"=w94) -> ()  [unwired: 10 in, 1 out]
                n132 = call-poly <vilib>:"Delacor_lib_QMH_Enqueue Message (poly).vi"("Message Data"=TRUE, "Message"="Panel Status" ("format string"), "Message Queue in"=w90) -> ("error out"=w95:errorcluster)  [unwired: 7 in, 1 out]
                n133 = call "Status Updated.vi"("Status"="Panel shown." ("format string"), "Module ID"=w91) -> ()  [unwired: 9 in, 1 out]
              }
            }
          }
          event User Event {
            # "Another Module called the \"Hide Panel\" API Method."
            n134 = event-data() -> ("Module ID"=w98:i32)  [unwired: 1 in]
            n135 = call "Addressed to This Module.vi"("Module ID from Argument"=w98, "Module Admin"=w97) -> ("Addressed to this instance?"=w99:bool)  [unwired: 8 in, 1 out]
            n136 = case shown="True" w99 {
              tunnel: w97 -> [_ w105]
              tunnel: w96 -> [_ w101]
              tunnel: [_ w108] -> w100
              frame False {
              }
              frame True {
                n137 = control-ref of="This VI"() -> (w107:refnum<vi>)
                n138 = property class="Mod Admin"(reference=w105) -> ("Accessors:Module ID"=w104:i32)  [unwired: 1 in, 2 out]
                n139 = call "Hide VI Panel.vi"("VI"=w107) -> ()  [unwired: 10 in, 1 out]
                n140 = call "Status Updated.vi"("Status"="Panel hidden." ("format string"), "Module ID"=w104) -> ()  [unwired: 9 in, 1 out]
                n141 = call-poly <vilib>:"Delacor_lib_QMH_Enqueue Message (poly).vi"("Message Data"=FALSE, "Message"="Panel Status" ("format string"), "Message Queue in"=w101) -> ("error out"=w108:errorcluster)  [unwired: 7 in, 1 out]
              }
            }
          }
          event User Event {
            # "For cloneable running as singleton, broadcast that the module is running."
            n142 = event-data() -> ("Module ID"=w109:i32)  [unwired: 1 in]
            n143 = call "Addressed to This Module.vi"("Module ID from Argument"=w109, "Module Admin"=w110) -> ("Addressed to this instance?"=w111:bool)  [unwired: 8 in, 1 out]
            n144 = case shown="True" w111 {
              tunnel: [_ w115] -> w112
              tunnel: w109 -> [_ w114]
              frame False {
              }
              frame True {
                n145 = call "Update Module Execution Status.vi"("Running?"=TRUE, "Module ID"=w114) -> ("error out"=w115:errorcluster)  [unwired: 9 in]
              }
            }
          }
          event User Event {
            # "Another Module called the \"Show Diagram\" API Method. This event is used for debugging."
            n146 = event-data() -> ("Module ID"=w117:i32)  [unwired: 1 in]
            n147 = call "Addressed to This Module.vi"("Module ID from Argument"=w117, "Module Admin"=w116) -> ("Addressed to this instance?"=w118:bool)  [unwired: 8 in, 1 out]
            n148 = case shown="True" w118 {
              tunnel: w116 -> [_ w119]
              frame False {
              }
              frame True {
                n149 = disable-structure shown="RUN_TIME_ENGINE==False" {
                  disable-tunnel: w119 -> [w120 _]
                  frame condition #0 (active) {
                    # "functionality not available in exe"
                    n150 = invoke class="VI" method="Lock State.Get"() -> (error out=w126:errorcluster, "Get Lock State"=w125:T5, "pwd in cache"=w122:bool)  [unwired: 4 in, 1 out]
                    n151 = Equal?(x=T5."Password-protected", y=w125) -> (x = y?=w123:bool)
                    n152 = Compound Arithmetic op=AND(w123, invert w122) -> (w121:bool)
                    n153 = case shown="False" w121 {
                      tunnel: w126 -> [w131 _]
                      tunnel: w120 -> [w128 _]
                      frame False {
                        n154 = property class="Mod Admin"(reference=w128) -> ("Accessors:Module ID"=w127:i32)  [unwired: 1 in, 2 out]
                        n155 = property class="VI"(error in=w131, "BDWin.Open"=TRUE ("Block Diagram Window:Open")) -> ()  [unwired: 1 in, 2 out]
                        n156 = call "Status Updated.vi"("Status"="Block Diagram shown." ("format string"), "Module ID"=w127) -> ()  [unwired: 9 in, 1 out]
                      }
                      frame True {
                        # "Password-protected VI, and the password is not in the cache. Do not show the diagram."
                      }
                    }
                  }
                  frame condition #1 {
                  }
                }
              }
            }
          }
          event User Event {
            # "Another Module called the \"Stop Module\" API Method  or the Message Handling Loop below."
            n157 = event-data() -> ("Module ID"=w133:i32, "Wait for Module to stop?"=w134:bool, "Origin"=w132:string)  [unwired: 1 in]
            n158 = call "Addressed to This Module.vi"("Module ID from Argument"=w133, "Module Admin"=w137) -> ("Addressed to this instance?"=w136:bool)  [unwired: 8 in, 1 out]
            n159 = case shown="True" w136 {
              tunnel: [_ w151] -> w139
              tunnel: w138 -> [_ w147]
              tunnel: [_ TRUE] -> w135
              tunnel: w134 -> [_ w142]
              tunnel: w133 -> [_ w144]
              tunnel: w132 -> [_ w140]
              frame False {
              }
              frame True {
                # "The event can get fired from the Exit message. The queue gets destroyed there. In this case, the Enqueue VI will return error 1. It is safe to ignore, because the module is already exiting."
                n160 = local write "Status"(w140) -> ()
                n161 = Bundle By Name(cluster=T6 {"Module ID"=-1, "Origin"="", "Exit via Stop Module Req?"=FALSE, "Wait for Module to stop?"=FALSE} ("Stop Argument"), "Module ID"=w144, "Exit via Stop Module Req?"=TRUE, "Wait for Module to stop?"=w142) -> (w141:T6)
                n162 = call-poly <vilib>:"Delacor_lib_QMH_Enqueue Message (poly).vi"("Priority Message? (F)"=TRUE, "Message Data"=w141, "Message"="Exit", "Message Queue in"=w147) -> ("error out"=w152:errorcluster)  [unwired: 6 in, 1 out]
                n163 = call <vilib>:"Clear Errors.vi"("error in (no error)"=w152, "specific error code to clear (0: all)"=1) -> ("error out"=w151:errorcluster)  [unwired: 4 in, 1 out]
              }
            }
          }
          event Panel Close? {
            w156 = TRUE  # Discard the event, the MHL is responsible for closing and stopping this VI.
            # "Hide the panel or send the 'Exit' message if the user clicks the 'X' on the module main VI panel."
            n164 = event-data() -> ()  [unwired: 1 in, 1 out]
            n165 = property class="Mod Admin"(reference=w155) -> ("Accessors:External Launch"=w153:bool)  [unwired: 1 in, 2 out]
            n166 = case shown="True" w153 {
              tunnel: w154 -> [_ w161]
              tunnel: [_ w162] -> w157
              frame True {
                # "If externally launched, clicking the 'X' hides the panel, but doesn't close it."
                n167 = control-ref of="This VI"() -> (w158:refnum<vi>)
                n168 = call "Hide VI Panel.vi"("VI"=w158) -> ()  [unwired: 10 in, 1 out]
              }
              frame False {
                # "If run as a stand-alone VI, clicking the panel 'X' stops the VI."
                n169 = call-poly <vilib>:"Delacor_lib_QMH_Enqueue Message (poly).vi"("Priority Message? (F)"=TRUE, "Message"="Exit", "Message Queue in"=w161) -> ("error out"=w162:errorcluster)  [unwired: 7 in, 1 out]
              }
            }
            n170 = event-data("Discard?"=w156) -> ()  [unwired: 1 in, 1 out]
          }
          event User Event {
            # "Another Module called the \"Draw Panel into Subpanel\" API Method."
            n171 = event-data() -> ("Module ID"=w164:i32, "Sub Panel"=w163:refnum<vi>)  [unwired: 1 in]
            n172 = Bundle(cluster=T7 {"Module ID"=-1, "Sub Panel"=refnum} ("Draw Panel into Subpanel Argument"), "Module ID"=w164, "Sub Panel"=w163) -> (w165:T7)
            n173 = call "Addressed to This Module.vi"("Module ID from Argument"=w164, "Module Admin"=w167) -> ("Addressed to this instance?"=w168:bool)  [unwired: 8 in, 1 out]
            n174 = case shown="True" w168 {
              tunnel: w169 -> [_ w173]
              tunnel: w165 -> [_ w171]
              tunnel: [_ w174] -> w170
              frame False {
              }
              frame True {
                n175 = call-poly <vilib>:"Delacor_lib_QMH_Enqueue Message (poly).vi"("Message Data"=w171, "Message"="Draw Panel into Subpanel", "Message Queue in"=w173) -> ("error out"=w174:errorcluster)  [unwired: 7 in, 1 out]
              }
            }
          }
          event User Event {
            # "Another Module called the \"Remove Panel from Subpanel\" API Method."
            n176 = event-data() -> ("Module ID"=w176:i32, "Boolean"=w175:bool)  [unwired: 1 in]
            n177 = Bundle(cluster=T8 {"Module ID"=-1, "Boolean"=FALSE} ("Remove Panel from Subpanel Argument"), "Module ID"=w176, "Boolean"=w175) -> (w177:T8)
            n178 = call "Addressed to This Module.vi"("Module ID from Argument"=w176, "Module Admin"=w179) -> ("Addressed to this instance?"=w180:bool)  [unwired: 8 in, 1 out]
            n179 = case shown="True" w180 {
              tunnel: w181 -> [_ w185]
              tunnel: w177 -> [_ w183]
              tunnel: [_ w186] -> w182
              frame False {
              }
              frame True {
                n180 = call-poly <vilib>:"Delacor_lib_QMH_Enqueue Message (poly).vi"("Message Data"=w183, "Message"="Remove Panel from Subpanel", "Message Queue in"=w185) -> ("error out"=w186:errorcluster)  [unwired: 7 in, 1 out]
              }
            }
          }
          event User Event {
            # "Another Module called the \"Connect\" API Method."
            n181 = event-data() -> ("Module ID"=w189:i32, "VISA resource"=w188:refnum<visa-resource-name>)  [unwired: 1 in]
            n182 = Bundle(cluster=T9 {"Module ID"=-1, "VISA resource"=""} ("Connect Argument"), "Module ID"=w189, "VISA resource"=w188) -> (w190:T9)
            n183 = call "Addressed to This Module.vi"("Module ID from Argument"=w189, "Module Admin"=w192) -> ("Addressed to this instance?"=w193:bool)  [unwired: 8 in, 1 out]
            n184 = case shown="True" w193 {
              tunnel: w194 -> [_ w198]
              tunnel: w190 -> [_ w196]
              tunnel: [_ w195] -> w187
              frame False {
              }
              frame True {
                n185 = call-poly <vilib>:"Delacor_lib_QMH_Enqueue Message (poly).vi"("Message Data"=w196, "Message"="Connect", "Message Queue in"=w198) -> ("error out"=w195:errorcluster)  [unwired: 7 in, 1 out]
              }
            }
          }
          event User Event {
            # "Another Module called the \"Disconnect\" API Method."
            n186 = event-data() -> ("Module ID"=w201:i32, "Boolean"=w200:bool)  [unwired: 1 in]
            n187 = Bundle(cluster=T10 {"Module ID"=-1, "Boolean"=FALSE} ("Disconnect Argument"), "Module ID"=w201, "Boolean"=w200) -> (w202:T10)
            n188 = call "Addressed to This Module.vi"("Module ID from Argument"=w201, "Module Admin"=w204) -> ("Addressed to this instance?"=w205:bool)  [unwired: 8 in, 1 out]
            n189 = case shown="True" w205 {
              tunnel: w206 -> [_ w210]
              tunnel: w202 -> [_ w208]
              tunnel: [_ w207] -> w199
              frame False {
              }
              frame True {
                n190 = call-poly <vilib>:"Delacor_lib_QMH_Enqueue Message (poly).vi"("Message Data"=w208, "Message"="Disconnect", "Message Queue in"=w210) -> ("error out"=w207:errorcluster)  [unwired: 7 in, 1 out]
              }
            }
          }
          event User Event {
            # "Another Module called the \"Configure\" API Method."
            n191 = event-data() -> ("Module ID"=w214:i32, "Acquisition type"=w211:enum16{"On demand", "Continous"}, "Config parameters"=w212:T12)  [unwired: 1 in]
            n192 = Bundle(cluster=T11 {"Module ID"=-1, "Acquisition type"=enum."On demand", "Config parameters"={"Acquisition Type"=0, "Averaged Waveforms"=4, "Channel"=0, "Probe Attenuation"=10, "Timebase"=0.0}} ("Configure Argument"), "Module ID"=w214, "Acquisition type"=w211, "Config parameters"=w212) -> (w215:T11)
            n193 = call "Addressed to This Module.vi"("Module ID from Argument"=w214, "Module Admin"=w217) -> ("Addressed to this instance?"=w218:bool)  [unwired: 8 in, 1 out]
            n194 = case shown="True" w218 {
              tunnel: w219 -> [_ w223]
              tunnel: w215 -> [_ w221]
              tunnel: [_ w220] -> w213
              frame False {
              }
              frame True {
                n195 = call-poly <vilib>:"Delacor_lib_QMH_Enqueue Message (poly).vi"("Message Data"=w221, "Message"="Configure acquisition", "Message Queue in"=w223) -> ("error out"=w220:errorcluster)  [unwired: 7 in, 1 out]
              }
            }
          }
          event User Event {
            # "Another Module called the \"Configure trigger\" API Method."
            n196 = event-data() -> ("Module ID"=w226:i32, "Trigger config"=w224:T14)  [unwired: 1 in]
            n197 = Bundle(cluster=T13 {"Module ID"=-1, "Trigger config"={"Trigger Source"=0, "Trigger Mode"=0, "Trigger Slope"=0, "Trigger Coupling"=0, "Trigger Level"=0.0}} ("Configure trigger Argument"), "Module ID"=w226, "Trigger config"=w224) -> (w227:T13)
            n198 = call "Addressed to This Module.vi"("Module ID from Argument"=w226, "Module Admin"=w229) -> ("Addressed to this instance?"=w230:bool)  [unwired: 8 in, 1 out]
            n199 = case shown="True" w230 {
              tunnel: w231 -> [_ w235]
              tunnel: w227 -> [_ w233]
              tunnel: [_ w232] -> w225
              frame False {
              }
              frame True {
                n200 = call-poly <vilib>:"Delacor_lib_QMH_Enqueue Message (poly).vi"("Message Data"=w233, "Message"="Configure trigger", "Message Queue in"=w235) -> ("error out"=w232:errorcluster)  [unwired: 7 in, 1 out]
              }
            }
          }
          event User Event {
            # "Another Module called the \"Send software trigger\" API Method."
            n201 = event-data() -> ("Module ID"=w238:i32, "Boolean"=w237:bool)  [unwired: 1 in]
            n202 = Bundle(cluster=T15 {"Module ID"=-1, "Boolean"=FALSE} ("Send software trigger Argument"), "Module ID"=w238, "Boolean"=w237) -> (w239:T15)
            n203 = call "Addressed to This Module.vi"("Module ID from Argument"=w238, "Module Admin"=w241) -> ("Addressed to this instance?"=w242:bool)  [unwired: 8 in, 1 out]
            n204 = case shown="True" w242 {
              tunnel: w243 -> [_ w247]
              tunnel: w239 -> [_ w245]
              tunnel: [_ w244] -> w236
              frame False {
              }
              frame True {
                n205 = call-poly <vilib>:"Delacor_lib_QMH_Enqueue Message (poly).vi"("Message Data"=w245, "Message"="Send software trigger", "Message Queue in"=w247) -> ("error out"=w244:errorcluster)  [unwired: 7 in, 1 out]
              }
            }
          }
          event User Event {
            # "Another Module called the \"Start continuous acquistion\" API Method."
            n206 = event-data() -> ("Module ID"=w250:i32, "Timeout"=w249:i32)  [unwired: 1 in]
            n207 = Bundle(cluster=T16 {"Module ID"=-1, "Timeout"=0} ("Start continuous acquistion Argument"), "Module ID"=w250, "Timeout"=w249) -> (w251:T16)
            n208 = call "Addressed to This Module.vi"("Module ID from Argument"=w250, "Module Admin"=w253) -> ("Addressed to this instance?"=w254:bool)  [unwired: 8 in, 1 out]
            n209 = case shown="True" w254 {
              tunnel: w255 -> [_ w259]
              tunnel: w251 -> [_ w257]
              tunnel: [_ w256] -> w248
              frame False {
              }
              frame True {
                n210 = call-poly <vilib>:"Delacor_lib_QMH_Enqueue Message (poly).vi"("Message Data"=w257, "Message"="Start continuous acquistion", "Message Queue in"=w259) -> ("error out"=w256:errorcluster)  [unwired: 7 in, 1 out]
              }
            }
          }
          event User Event {
            # "Another Module called the \"Stop continuous acquisition\" API Method."
            n211 = event-data() -> ("Module ID"=w262:i32, "Boolean"=w261:bool)  [unwired: 1 in]
            n212 = Bundle(cluster=T17 {"Module ID"=-1, "Boolean"=FALSE} ("Stop continuous acquisition Argument"), "Module ID"=w262, "Boolean"=w261) -> (w263:T17)
            n213 = call "Addressed to This Module.vi"("Module ID from Argument"=w262, "Module Admin"=w265) -> ("Addressed to this instance?"=w266:bool)  [unwired: 8 in, 1 out]
            n214 = case shown="True" w266 {
              tunnel: w267 -> [_ w271]
              tunnel: w263 -> [_ w269]
              tunnel: [_ w268] -> w260
              frame False {
              }
              frame True {
                n215 = call-poly <vilib>:"Delacor_lib_QMH_Enqueue Message (poly).vi"("Message Data"=w269, "Message"="Stop continuous acquisition", "Message Queue in"=w271) -> ("error out"=w268:errorcluster)  [unwired: 7 in, 1 out]
              }
            }
          }
          event User Event {
            # "Another Module called the \"Get measurement\" API Method."
            n216 = event-data() -> ("Module ID"=w277:i32, "Channel"=w276:i32, "Measurement Type"=w275:i32, "Wait Notifier"=w274:refnum<notifier>, "wait for reply"=w273:bool)  [unwired: 1 in]
            n217 = Bundle(cluster=T18 {"Module ID"=-1, "Channel"=1, "Measurement Type"=0, "Wait Notifier"=refnum, "wait for reply"=FALSE} ("Get measurement Argument"), "Module ID"=w277, "Channel"=w276, "Measurement Type"=w275, "Wait Notifier"=w274, "wait for reply"=w273) -> (w278:T18)
            n218 = call "Addressed to This Module.vi"("Module ID from Argument"=w277, "Module Admin"=w280) -> ("Addressed to this instance?"=w281:bool)  [unwired: 8 in, 1 out]
            n219 = case shown="True" w281 {
              tunnel: w282 -> [_ w286]
              tunnel: w278 -> [_ w284]
              tunnel: [_ w283] -> w272
              frame False {
              }
              frame True {
                n220 = call-poly <vilib>:"Delacor_lib_QMH_Enqueue Message (poly).vi"("Message Data"=w284, "Message"="Get measurement", "Message Queue in"=w286) -> ("error out"=w283:errorcluster)  [unwired: 7 in, 1 out]
              }
            }
          }
          event User Event {
            # "Another Module called the \"Configure timebase\" API Method."
            n221 = event-data() -> ("Module ID"=w289:i32, "Timebase"=w288:dbl)  [unwired: 1 in]
            n222 = Bundle(cluster=T19 {"Module ID"=-1, "Timebase"=0.0005} ("Configure timebase Argument"), "Module ID"=w289, "Timebase"=w288) -> (w290:T19)
            n223 = call "Addressed to This Module.vi"("Module ID from Argument"=w289, "Module Admin"=w292) -> ("Addressed to this instance?"=w293:bool)  [unwired: 8 in, 1 out]
            n224 = case shown="True" w293 {
              tunnel: w294 -> [_ w298]
              tunnel: w290 -> [_ w296]
              tunnel: [_ w295] -> w287
              frame False {
              }
              frame True {
                n225 = call-poly <vilib>:"Delacor_lib_QMH_Enqueue Message (poly).vi"("Message Data"=w296, "Message"="Configure timebase", "Message Queue in"=w298) -> ("error out"=w295:errorcluster)  [unwired: 7 in, 1 out]
              }
            }
          }
        }
        n226 = call-dynamic "Delacor_lib_QMH_Error Handler - Event Handling Loop.vi"("error in"=w82, "Message Queue in"=w76) -> ("dup error in"=w81:errorcluster)  [unwired: 8 in, 1 out]
      }
      n227 = while {
        tunnel: w29 -> [w45]
        tunnel: w31 -> [w49]
        shift-right: [w47] -> _
        shift-left: -1 ("Helper Loop Timeout") -> [w48]
        tunnel: [w46] -> w32
        tunnel: [w51] -> w37
        tunnel: w28 -> [w43]
        shift-right: [w42] -> _
        shift-left: _ -> [w41]
        stop <- w44 stop-if-true
        # "Helper Loop"
        n228 = event shown="[2] <Local Events.Wake up Helper Loop>: User Event" {
          selector: w49 -> [_ _ _ _]
          dyn-events: [_ _ _ _] -> w46
          timeout: w48 -> [_ _ _ _]
          tunnel: w48 -> [w58 w63 _ _]
          tunnel: [w58 w63 w66 -1 ("Helper Loop Timeout")] -> w47
          tunnel: [_ w60 _ _] -> w44
          tunnel: w43 -> [w56 w62 w64 w74]
          tunnel: [w57 _ w69 w75] -> w50
          tunnel: [w53 w59 w65 w70] -> w42
          tunnel: w41 -> [w53 w59 _ w70]
          event Timeout {
            # "Continuous Tasks"
            n229 = event-data() -> ()  [unwired: 1 in, 1 out]
            n230 = call-poly <instrlib>:"Read.vi"("VISA resource name"=w53) -> ("error out"=w54:errorcluster, "Waveform Data"=w52:waveform(dbl))  [unwired: 8 in, 1 out]
            n231 = property class="Mod Admin"(reference=w56) -> ("Accessors:Module ID"=w55:i32)  [unwired: 1 in, 2 out]
            n232 = call "Data acquired.vi"("error in"=w54, "Waveform"=w52, "Module ID"=w55) -> ("error out"=w57:errorcluster)  [unwired: 8 in]
            n233 = local write "Waveform Data"(w52) -> ()
          }
          event User Event {
            # "If Request is addressed for\nthis module instance then Stop Helper Loop"
            # "Helper Loop Suscribed to DQMH Stop Module Request"
            n234 = event-data() -> ("Module ID"=w61:i32)  [unwired: 1 in]
            n235 = call "Addressed to This Module.vi"("Module ID from Argument"=w61, "Module Admin"=w62) -> ("Addressed to this instance?"=w60:bool)  [unwired: 8 in, 1 out]
          }
          event User Event {
            # "Wake up Helper Loop, Start Continuous Tasks"
            n236 = event-data() -> ("Helper Loop Timeout"=w66:i32, "VISA resource name"=w65:refnum<visa-resource-name>)  [unwired: 1 in]
            n237 = property class="Mod Admin"(reference=w64) -> ("Accessors:Module ID"=w67:i32)  [unwired: 1 in, 2 out]
            n238 = call "Helper Loop Status Updated.vi"("Helper Loop Status"=Helper_Loop_Status--enum."Awake", "Module ID"=w67) -> ("error out"=w69:errorcluster)  [unwired: 9 in]
          }
          event User Event {
            # "#PantherLAB_How_To\nWhen Put Helper Loop to Sleep Private Request is executed\na new Helper Loop Timeout will be set to -1 meaning this\nHelper Loop will stop doing continuous tasks"
            # "Put Helper Loop to Sleep"
            n239 = event-data() -> ()  [unwired: 1 in, 1 out]
            n240 = property class="Mod Admin"(reference=w74) -> ("Accessors:Module ID"=w71:i32)  [unwired: 1 in, 2 out]
            n241 = call "Helper Loop Status Updated.vi"("Helper Loop Status"=Helper_Loop_Status--enum."Asleep", "Module ID"=w71) -> ("error out"=w75:errorcluster)  [unwired: 9 in]
          }
        }
        n242 = call-dynamic "Delacor_lib_QMH_Error Handler - Helper Loop.vi"("error in"=w50, "Message Queue in"=w45) -> ("dup error in"=w51:errorcluster)  [unwired: 8 in, 1 out]
      }
    }
    frame Error {
      n243 = call "Synchronize Caller Events.vi"("Module Admin"=w571) -> ("Module Admin out"=w570:refnum<class "Delacor_lib_QMH_Cloneable Module Admin.lvclass">)  [unwired: 9 in, 1 out]
      n244 = property class="Mod Admin"(reference=w570) -> ("Accessors:Module ID"=w569:i32)  [unwired: 1 in, 2 out]
      n245 = call-dynamic "Delacor_lib_QMH_Release Message Queue.vi"("error in"=w577, "Message Queue"=w568) -> ("error out"=w576:errorcluster)  [unwired: 9 in]
      n246 = call "Module Name--constant.vi"("Module ID"=w569) -> ("Module Name"=w574:string)  [unwired: 10 in]
      n247 = Format Into String(format string="An error occurred during initialization. %s is no longer running.", w574) -> (resulting string=w572:string)  [unwired: 2 in, 1 out]
      n248 = call "Error Reported.vi"("Additional Information"=w572, "Error"=w576, "Module ID"=w569) -> ()  [unwired: 8 in, 1 out]
    }
  }
  n249 = Merge Errors(w25, w24, w17) -> (w26:errorcluster)
  n250 = Unregister For Events(event registration refnum=w6) -> (error out=w15:errorcluster)  [unwired: 1 in]
  n251 = call "Close Module.vi"("error in"=w26, "Wait for stop?"=w8, "Module Admin in"=w10) -> ("error out"=w22:errorcluster, "External Launch"=w7:bool, "Module Admin out"=w9:refnum<class "Delacor_lib_QMH_Cloneable Module Admin.lvclass">)  [unwired: 6 in]
  n252 = call "Destroy Local Events.vi"("error in"=w15, "Local Events"=w1) -> ()  [unwired: 9 in, 1 out]
  n253 = Unregister For Events(event registration refnum=w14, error in=w22) -> (error out=w21:errorcluster)
  "error out" <- w21
  n254 = local write "Module Admin"(w9) -> ()
  n255 = case "External Launch?" shown="True" w7 {
    tunnel: w21 -> [_ w578]
    frame False {
    }
    frame True {
      n256 = case shown="No Error" w578 {
        frame No Error {
          n257 = invoke class="VI" method="FP.Close"() -> ()  [unwired: 3 in, 3 out]
        }
        frame Error {
          n258 = invoke class="VI" method="FP.Open"("Activate"=TRUE ("Activate?")) -> ()  [unwired: 4 in, 5 out]
        }
      }
    }
  }
